vi "PS35_CmdAnsEx.vi"(4 "error in (no error)":errorcluster, 6 "nBreak":i32 min=0, 7 "nRequest":i32 min=0 max=1, 8 "Command":string, 9 "Control unit ID":i32=1 min=1 max=10) -> (0 "error out":errorcluster, 1 "String length":i32, 2 "Answer string":string)   [LabVIEW 2020]
doc: "PS35_CmdAnsEx.vi, created: 14.06.2010 alex; last change: 22.10.2019 alex;\n\n<B>FUNCTION:</B> \n\nSend direct commands to the control unit (low level communication\nwith defined delay in ms).\nOne can communicate with this function with the control unit directly. \nThe commands from the command reference of the control unit are used.\nThe maximum size of the communication buffer is 100 characters.\n----------------------------------------------------------------------------------------\n<B>INPUT:</B>\n[I32] <B>Control unit ID:</B> control unit index. (Default=1, Range=1...10)\n[CStr] <B>Command:</B> command from the command reference. (Default=empty string) \n[I32] <B>nRequest:</B> request mode. (Default=0, Range=0...1)\n0 - send command to the control unit (no request),\n1 - send command and after that read answer.\n[I32] <B>nBreak:</B> delay value for communication (nBreak>0),\nelse the pre-setting value is used.\n[CLU] <B>error in</B>\n----------------------------------------------------------------------------------------\n<B>OUTPUT:</B>\n[CStr] <B>Answer string:</B> answer from the control unit.\n[I32] <B>String length:</B> length of the answer string.\n[CLU] <B>error out</B>\n----------------------------------------------------------------------------------------\n<B>SUB-VIs:</B>\nPS35_GetReadError.vi\n----------------------------------------------------------------------------------------\n<B>EXT-Calls:</B>\nps35.dll (V2.01)\n----------------------------------------------------------------------------------------"
uses:
  ps35.dll
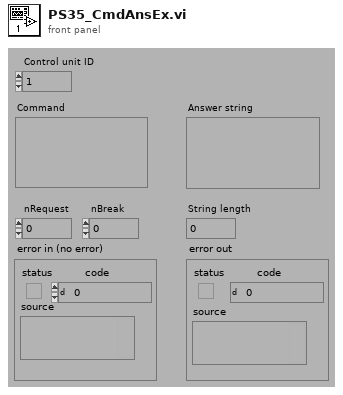
[diagram p1: front panel]
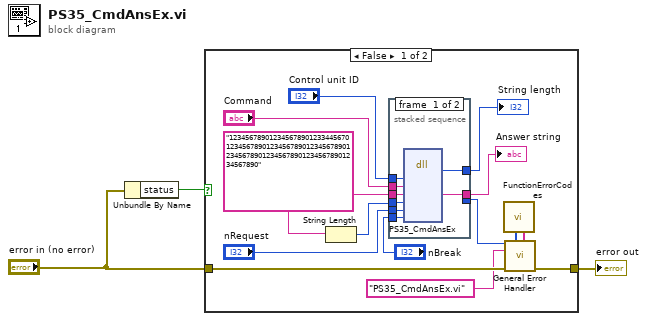
[diagram p0: block diagram]
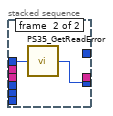
[diagram p2: hidden frame]
diagram:
  n1 = Unbundle By Name("error in (no error)") -> ("status"=w1:bool)
  n2 = case shown="False" w1 {
    tunnel: "error in (no error)" -> [w16 w28]
    tunnel: [w15 w28] -> w3
    frame False {
      w10 = "1234567890123456789012334456701234567890123456789012345678901234567890123456789012345678901234567890"
      n3 = String Length(string=w10) -> (length=w11:i32)
      n4 = stacked-sequence {
        tunnel: "Control unit ID" -> [w25 w27]
        tunnel: [w24 _] -> w14
        tunnel: [_ w26] -> w13
        tunnel: [w23 _] -> w12
        tunnel: w11 -> [w22 _]
        tunnel: w10 -> [w21 _]
        tunnel: "Command" -> [w20 _]
        tunnel: "nRequest" -> [w19 _]
        tunnel: "nBreak" -> [w18 _]
        frame #0 {
          n5 = dll-call lib="C:/GEECS/Developers Version/source/Device Drivers/OwiSoft/OWISoftOEM/ps35/labview/lv82/ps35.dll" fn="PS35_CmdAnsEx" label="PS35_\nCmdAnsEx"("Index"=w25, "szCmd"=w20, "szAns"=w21, "Length"=w22, "nRequest"=w19, "nBreak"=w18) -> ("Rückgabetyp"=w24:i32, "szAns"=w23:string)  [unwired: 8 in, 2 out]
        }
        frame #1 {
          n6 = call "PS35_GetReadError.vi"("Control unit ID"=w27) -> ("Read error"=w26:i32)
        }
      }
      "Answer string" <- w12
      "String length" <- w14
      n7 = call "FunctionErrorCodes.vi"() -> ("[user-defined codes]"=w5:i32[], "[user-defined descriptions]"=w4:string[])  [unwired: 8 in]
      n8 = call <vilib>:"General Error Handler.vi"("[error code] (0)"=w13, "[user-defined codes]"=w5, "[user-defined descriptions]"=w4, "[error source] (\" \")"="PS35_CmdAnsEx.vi" ("[error source] (\" \")"), "error in (no error)"=w16) -> ("error out"=w15:errorcluster)  [unwired: 6 in, 4 out]
    }
    frame True {
    }
  }
  "error out" <- w3
